vi "ExTestReadingF32FromImageExample.vi"() -> ()   [LabVIEW 2010]
panel:
  out "Test 2d Array":sgl[][](array[numeric]) format="%.2f"
  out "Test 1d array":sgl[](array[numeric]) format="%.2f"
  out "Pixel Value u16":u16
  out "Pixel Value i32":i32
  out "Pixel Value f32":sgl format="%.2f"
  out "error out":errorcluster
  in  "error in (no error)":errorcluster
  # "ExTestReadingFromImageExample\nThis example shows how to pull the data out of the\nToolkit data handle into the LabView world.\nThis specific example shows it for 32 bit float.\nAfter running this example the right allows you to \nlook at ramp that was created."
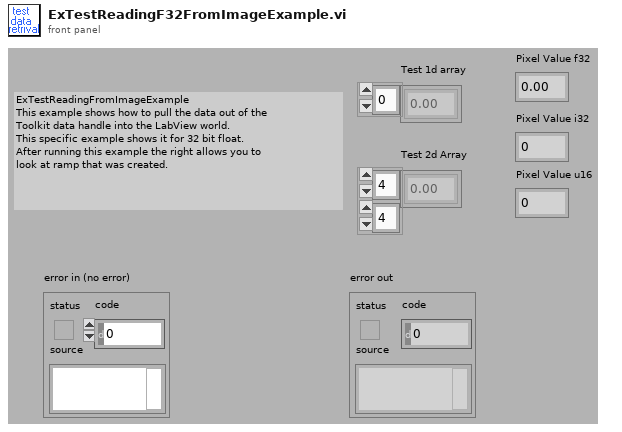
[diagram p1: front panel]
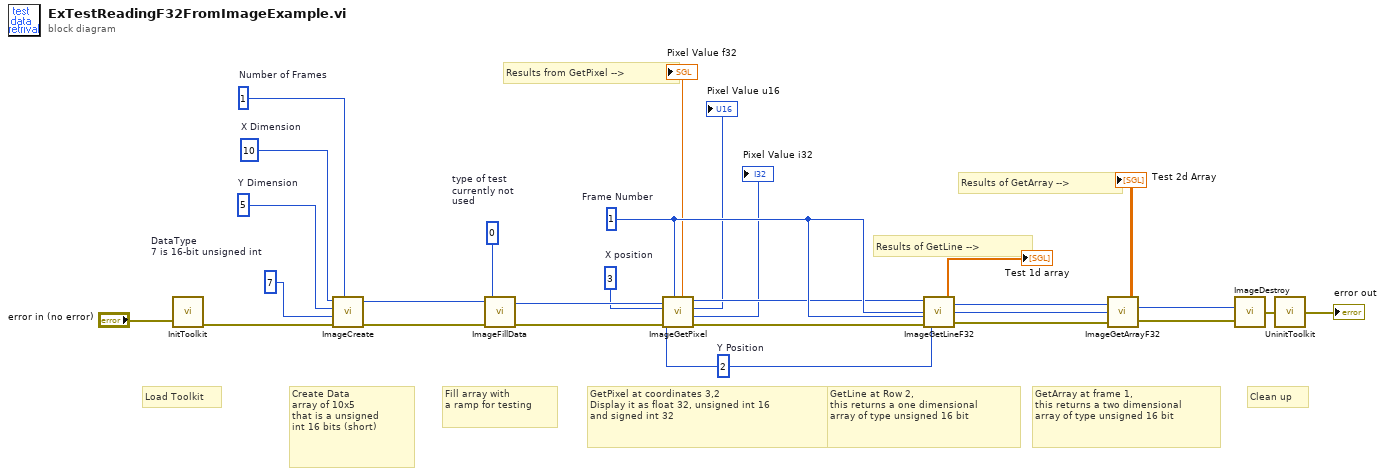
[diagram p0: block diagram]
diagram:
  w8 = 1  # Frame Number
  w11 = 2  # Y Position
  w12 = 3  # X position
  w14 = 0  # type of test currently not used
  w16 = 1  # Number of Frames
  w17 = 10  # X Dimension
  w18 = 5  # Y Dimension
  w19 = 7  # DataType  7 is 16-bit unsigned int
  # "Clean up"
  # "Results of GetArray -->"
  # "GetArray at frame 1,\nthis returns a two dimensional\narray of type unsigned 16 bit"
  # "GetLine at Row 2,\nthis returns a one dimensional\narray of type unsigned 16 bit"
  # "Results of GetLine -->"
  # "GetPixel at coordinates 3,2\nDisplay it as float 32, unsigned int 16\nand signed int 32"
  # "Results from GetPixel -->"
  # "Fill array with \na ramp for testing"
  # "Create Data\narray of 10x5\nthat is a unsigned \nint 16 bits (short)"
  # "Load Toolkit"
  n1 = call <userlib>:"InitToolkit.vi"("error in"="error in (no error)") -> ("error out"=w27:errorcluster)
  n2 = call <userlib>:"ImageCreate.vi"("X dimension"=w17, "Y dimension"=w18, "Data Type"=w19, "error in"=w27, "Number Of Frames"=w16) -> ("Image Handle"=w15:u32, "error out"=w23:errorcluster)
  n3 = call <userlib>:"ImageFillData.vi"("error in"=w23, "Type of Test"=w14, "Image Handle"=w15) -> ("error out"=w22:errorcluster, "Image Handle"=w13:u32)
  n4 = call <userlib>:"ImageGetPixel.vi"("Z position"=w8, "error in"=w22, "Y position"=w11, "X position"=w12, "Data Handle"=w13) -> ("error out"=w6:errorcluster, "Pixel Value i32"=→"Pixel Value i32":i32, "Pixel Value u16"=→"Pixel Value u16":u16, "Data Handle"=w7:u32, "Pixel Value f32"=→"Pixel Value f32":sgl)
  n5 = call <userlib>:"ImageGetLineF32.vi"("error in"=w6, "Z Position"=w8, "Y Position"=w11, "Data Handle"=w7) -> ("error out"=w21:errorcluster, "Array F32"=→"Test 1d array":sgl[], "Data Handle"=w10:u32)
  n6 = call <userlib>:"ImageGetArrayF32.vi"("error in"=w21, "Z position"=w8, "Image Handle"=w10) -> ("error out"=w20:errorcluster, "Array Float 32"=→"Test 2d Array":sgl[][], "Image Handle"=w9:u32)
  n7 = call <userlib>:"ImageDestroy.vi"("error in"=w20, "Data handle"=w9) -> ("error out"=w26:errorcluster)
  n8 = call <userlib>:"UninitToolkit.vi"("error in"=w26) -> ("error out"=→"error out":errorcluster)
